vi "Intake_Set.vi"   [LabVIEW 2019]
uses:
  Intake_States.ctl
  <vilib>/Rock Robotics/WPI/DriverStation/WPI_DriverStationRobotMode2.ctl
  Globals/Intake_Globals.vi
  Robot Global Data.vi
types:
  T1 = typedef "WPI_DriverStationRobotMode2.ctl" = enum16{"Autonomous Disabled", "Autonomous Enabled", "Teleop Disabled", "Teleop Enabled", "Disconnected", "Finish", "Test Disabled", "Test Enabled", "Emergency Stopped"}
  T2 = typedef "Intake_States.ctl" = enum16{"Manual_Control", "Compliant_Intake", "Command_RunIntake"}
  T3 = typedef "Intake_Cluster.ctl" = cluster{"Control_State":T2, "Intake_On":bool, "Intake_Extended":bool, "Intake_Throttle":dbl, "Auto_Notifier":refnum<notifier>, "Parameter_1":dbl, "Parameter_2":dbl, "Step":dbl, "Outtake":bool}
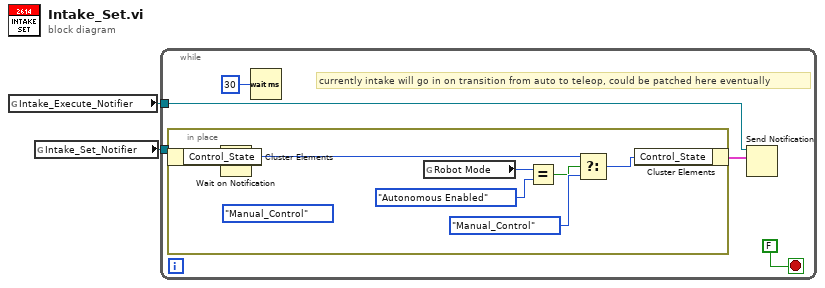
[diagram p0: block diagram]
diagram:
  n1 = global read "Intake_Globals.vi" "Intake_Execute_Notifier"() -> (w1:refnum<notifier>)
  n2 = global read "Intake_Globals.vi" "Intake_Set_Notifier"() -> (w2:refnum<notifier>)
  n3 = while {
    tunnel: w2 -> [w7]
    tunnel: w1 -> [w5]
    stop <- FALSE stop-if-true
    # "currently intake will go in on transition from auto to teleop, could be patched here eventually"
    n4 = Wait on Notification(notifier=w7) -> (notification=w6:T3)  [unwired: 3 in, 3 out]
    n5 = in-place {
      (unwired) Intake_States."Manual_Control" ("Control_State")
      n6 = in-place-cluster #1(w6) -> ("Control_State"=w9:T2)
      n7 = global read "Robot Global Data.vi" "Robot Mode"() -> (w12:T1)
      n8 = Equal?(x=w12, y=WPI_DriverStationRobotMode2."Autonomous Enabled") -> (x = y?=w10:bool)
      n9 = Select(t=w9, s=w10, f=Intake_States."Manual_Control" ("Control_State")) -> (s? t:f=w13:T2)
      n10 = in-place-cluster #1("Control_State"=w13) -> (w4:T3)
    }
    n11 = Wait (ms)(milliseconds to wait=u32 30) -> ()  [unwired: 1 out]
    n12 = Send Notification(notification=w4, notifier=w5) -> ()  [unwired: 1 in, 2 out]
  }
